vi "Polymorphic - Write and Read a Synchronous Message.vi"   [LabVIEW 2021]
doc: "Send a message and listen for the response. \n\nThe linefeed character is used to detect the end of the response message."
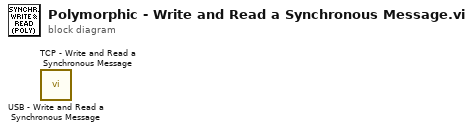
[diagram p0: block diagram]
diagram:
  n1 = call "USB - Write and Read a Synchronous Message.vi"() -> ()  [unwired: 9 in, 3 out]
  n2 = call "TCP - Write and Read a Synchronous Message.vi"() -> ()  [unwired: 9 in, 3 out]
